vi "GUI BPM RMS Min Max Monitoring Graph Window.vi"() -> ()   [LabVIEW 2011, in "User Interface Window VIs.lvlib"]
uses:
  User Interface Window VIs.lvlib
  Types Definitions/Type Monitoring Sample.ctl
  <vilib>/Platform/TimedLoop/XDataNode/timing_clust.ctl
  <vilib>/Platform/TimedLoop/XDataNode/nitl_modes.ctl
  <vilib>/Platform/TimedLoop/XDataNode/wakeup.ctl
  <vilib>/Analysis/5stat.llb/RMS (DBL).vi
  <vilib>/express/express shared/transition.llb/Dynamic To Waveform Array.vi
  <vilib>/express/express signal manip/GetorSetDDTAttributes/Set DDT Attributes/SetT0.vi
  <vilib>/express/express shared/transition.llb/Waveform Array To Dynamic.vi
  <vilib>/Platform/TimedLoop/XDataNode/XDataNode.xnode
  <vilib>/express/express signal manip/GetorSetDDTAttributes/Set DDT Attributes/Set DDT Properties.xnode
  <vilib>/Analysis/NI_AALPro.lvlib
  <vilib>/Platform/TimedLoop/XDataNode/XDNodeRunTimeDep.lvlib
  Type Definitions.lvlib
panel:
  out "Time Stamp on FOFB Controller":timestamp caption="Data/Hora Atual no\nControlador do FOFB"
  in  "All/None":bool=TRUE caption="Todos/Nenhum"
  out "Graph":dynamicdata(graph)=[{"t0"=timestamp(3442305362.414053 s since 1904-01-01), "dt"=1.0, "Y"=[0.6809232435425464], "attributes"=variant("NI_ExpTimeStamp"=variant(timestamp timestamp(3442305362.414053 s since 1904-01-01)))}, {"t0"=timestamp(3442305362.414053 s since 1904-01-01), "dt"=1.0, "Y"=[1.8957212522578981], "attributes"=variant("NI_ExpTimeStamp"=variant(timestamp timestamp(3442305362.414053 s since 1904-01-01)))}, {"t0"=timestamp(3442305362.414053 s since 1904-01-01), "dt"=1.0, "Y"=[0.04856006519213252], "attributes"=variant("NI_ExpTimeStamp"=variant(timestamp timestamp(3442305362.414053 s since 1904-01-01)))}, {"t0"=timestamp(3442305362.414053 s since 1904-01-01), "dt"=1.0, "Y"=[0.5450159966663619], "attributes"=variant("NI_ExpTimeStamp"=variant(timestamp timestamp(3442305362.414053 s since 1904-01-01)))}, {"t0"=timestamp(3442305362.414053 s since 1904-01-01), "dt"=1.0, "Y"=[1.4720034670901994], "attributes"=variant("NI_ExpTimeStamp"=variant(timestamp timestamp(3442305362.414053 s since 1904-01-01)))}, {"t0"=timestamp(3442305362.414053 s since 1904-01-01), "dt"=1.0, "Y"=[0.0014319434180204427], "attributes"=variant("NI_ExpTimeStamp"=variant(timestamp timestamp(3442305362.414053 s since 1904-01-01)))}]
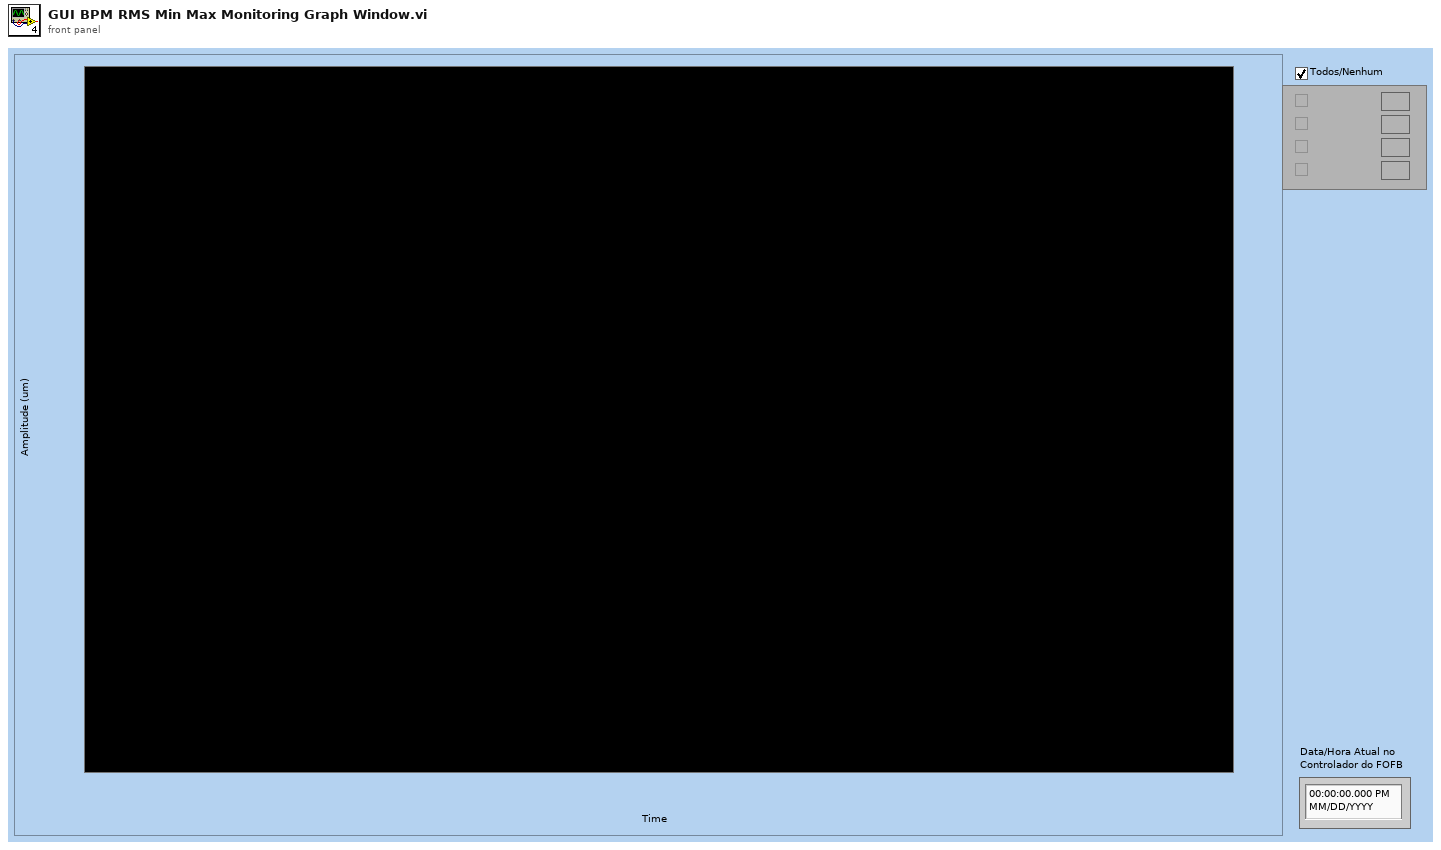
[diagram p1: front panel]
types:
  T1 = typedef "Type Definitions.lvlib/Type Monitoring Sample.ctl" = cluster{"Timestamp":timestamp, "Sample":dbl[]}
  T2 = typedef "XDNodeRunTimeDep.lvlib/timing_clust.ctl" = cluster{"Expected End [f-1]":u64, "Actual End [f-1]":u64, "Finished Late? [f-1]":bool, "Expected End [i-1]":u64, "Actual End [i-1]":u64, "Finished Late? [i-1]":bool, "Expected Start [i]":u64, "Actual Start [i]":u64, "Expected Start [f]":u64, "Actual Start [f]":u64, "Source Name":string, "Structure Name":string, "Period":i64, "Deadline":i64, "Offset":i64, "Start":i64, "Priority":i32, "Timeout":i32, "Mode":T3, "Wakeup Reason":T4, "Error":errorcluster, "Source Type":string, "Secondary Source Type":string, "Global End Time":u64, "Global Start Time":u64, "Frame Duration":u64, "Iteration Duration":u64, "Assigned CPU":i32, "I/O Scan Engine Mode":u32}
  T3 = typedef "XDNodeRunTimeDep.lvlib/nitl_modes.ctl" = enum32{"No Change", "Process missed periods, maintain original phase", "Discard missed periods, maintain original phase", "Process missed periods, ignore original phase", "Discard missed periods, ignore original phase"}
  T4 = typedef "XDNodeRunTimeDep.lvlib/wakeup.ctl" = enum32{"Normal", "Aborted", "Asynchronous wakeup", "Timing source error", "Timed loop error", "Timeout"}
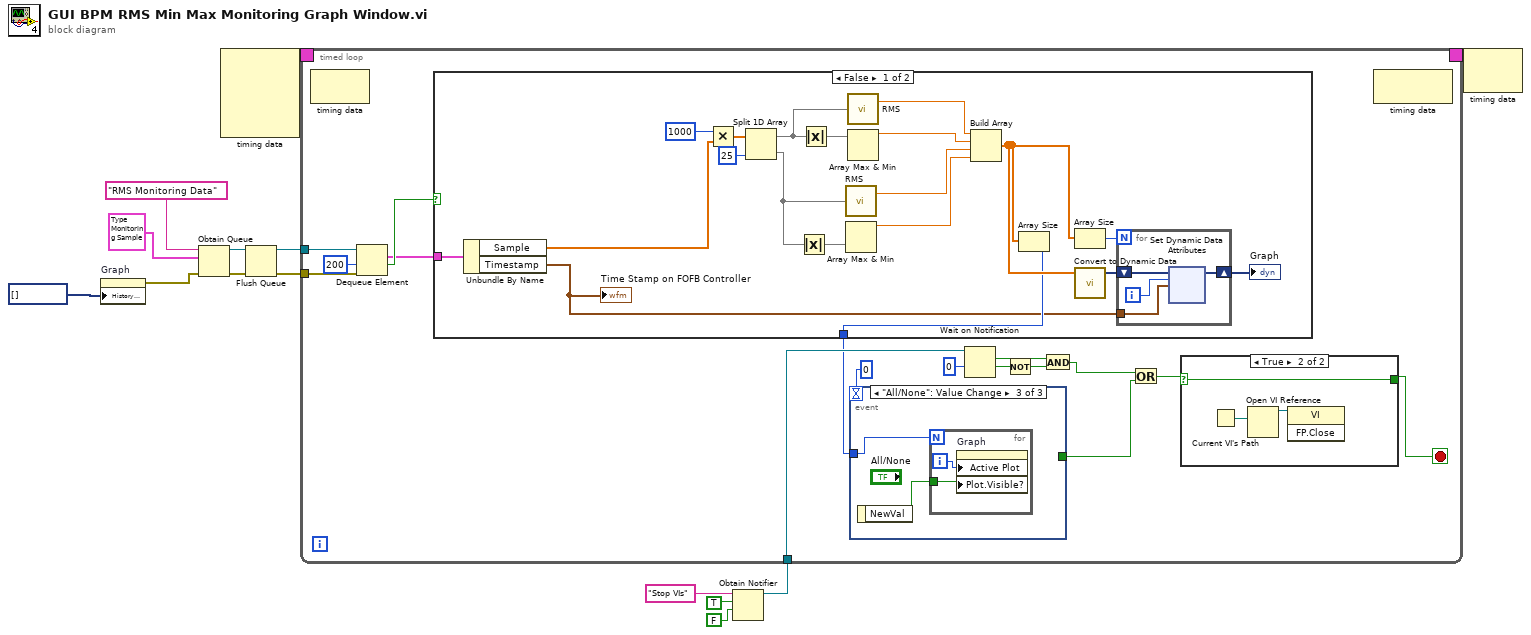
[diagram p0: block diagram]
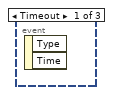
[diagram p4: hidden frame]
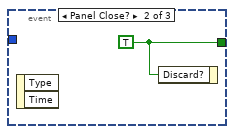
[diagram p5: hidden frame]
diagram:
  n1 = property on="Graph" class="WFChart (strict)"("History Data"=dynamicdata[] []) -> (error out=w5:errorcluster)  [unwired: 2 in, 1 out]
  n2 = Obtain Queue(name (unnamed)="RMS Monitoring Data", element data type=T1 {"Timestamp"=timestamp(0 s since 1904-01-01), "Sample"=[]} ("Monitoring Sample"), error in (no error)=w5) -> (queue out=w1:refnum<queue>, error out=w4:errorcluster)  [unwired: 2 in, 1 out]
  n3 = node-c288() -> (w14:T2)  [unwired: 4 in]
  n4 = Flush Queue(queue=w1, error in (no error)=w4) -> (queue out=w2:refnum<queue>, error out=w3:errorcluster)  [unwired: 1 out]
  n5 = Obtain Notifier(name (unnamed)="Stop VIs", notification data type=TRUE, create if not found? (T)=FALSE) -> (notifier out=w7:refnum<notifier>)  [unwired: 1 in, 2 out]
  n6 = timed-loop {
    timing: w14 -> [_]
    timing-out: [_] -> w13
    tunnel: w2 -> [w21]
    tunnel: w3 -> [w20]
    tunnel: w7 -> [w18]
    stop <- w22 stop-if-true
    n7 = node-c288() -> ()  [unwired: 1 in, 1 out]
    n8 = Dequeue Element(queue=w21, timeout in ms (-1)=200, error in (no error)=w20) -> (element=w15:T1, timed out?=w16:bool)  [unwired: 2 out]
    n9 = case shown="False" w16 {
      tunnel: [w34 _] -> w17
      tunnel: w15 -> [w33 _]
      frame False {
        n10 = Unbundle By Name(w33) -> ("Sample"=w32:dbl[], "Timestamp"=w31:timestamp)
        "Time Stamp on FOFB Controller" <- w31
        n11 = Multiply(x=1000, y=w32) -> (x*y=w39:dbl[])
        n12 = Split 1D Array(array=w39, index=25) -> (first subarray=w38:dbl[], second subarray=w37:dbl[])
        n13 = Absolute Value(x=w37) -> (abs(x)=w42:dbl[])
        n14 = Absolute Value(x=w38) -> (abs(x)=w43:dbl[])
        n15 = call-poly <vilib>:"RMS.vi"("X"=w37) -> ("rms value"=w41:dbl)  [unwired: 1 out]
        n16 = Array Max & Min(array=w42) -> (max value=w40:dbl)  [unwired: 3 out]
        n17 = call-poly <vilib>:"RMS.vi"("X"=w38) -> ("rms value"=w46:dbl)  [unwired: 1 out]
        n18 = Array Max & Min(array=w43) -> (max value=w45:dbl)  [unwired: 3 out]
        n19 = Build Array(w46, w45, w41, w40) -> (w35:dbl[])
        n20 = Array Size(array=w35) -> (size(s)=w34:i32)
        n21 = Array Size(array=w35) -> (size(s)=w49:i32)
        n22 = call "Convert to Dynamic Data"("Array"=w35) -> ("Dynamic Data Type"=w48:dynamicdata)  [unwired: 3 in]
        n23 = for {
          N: w49 -> [_]
          shift-right: [w53] -> w47
          shift-left: w48 -> [w51]
          tunnel: w31 -> [w50]
          i -> [w52]
          n24 = xnode ("Set Dynamic Data Attributes")("Signals In"=w51, "Signal Index"=w52, "Timestamp"=w50) -> ("Signals Out"=w53:dynamicdata)  [unwired: 1 in, 1 out]
        }
        "Graph" <- w47
      }
      frame True {
      }
    }
    n25 = event shown="[2] \"All/None\": Value Change" {
      selector: _ -> [_ _ _]
      dyn-events: _ -> [_ _ _]
      timeout: 0 -> [_ _ _]
      tunnel: [_ w71 _] -> w29
      tunnel: w17 -> [_ _ w72]
      event Timeout {
        n26 = event-data() -> ()  [unwired: 1 in, 2 out]
      }
      event Panel Close? {
        w71 = TRUE
        n27 = event-data() -> ()  [unwired: 1 in, 2 out]
        n28 = event-data("Discard?"=w71) -> ()  [unwired: 1 in, 1 out]
      }
      event "All/None": Value Change {
        n29 = event-data() -> ("NewVal"=w73:bool)  [unwired: 1 in]
        n30 = for {
          N: w72 -> [_]
          tunnel: w73 -> [w75]
          i -> [w74]
          n31 = property on="Graph" class="WFChart (strict)"("Active Plot"=w74, "Plot.Visible?"=w75) -> ()  [unwired: 2 in, 2 out]
        }
      }
    }
    n32 = Wait on Notification(notifier=w18, timeout in ms (-1)=0) -> (notification=w28:bool, timed out?=w26:bool)  [unwired: 2 in, 2 out]
    n33 = Not(x=w26) -> (.not. x?=w27:bool)
    n34 = And(x=w28, y=w27) -> (x .and. y?=w24:bool)
    n35 = Or(x=w24, y=w29) -> (x .or. y?=w23:bool)
    n36 = case shown="True" w23 {
      selector: w23 -> [w67 w69]
      tunnel: [w67 w69] -> w22
      frame False {
      }
      frame True {
        n37 = Current VI's Path() -> (path=w68:path)
        n38 = Open VI Reference(vi path=w68) -> (vi reference=w70:refnum<vi>)  [unwired: 5 in, 1 out]
        n39 = invoke class="VI" method="FP.Close"(reference=w70) -> ()  [unwired: 2 in, 3 out]
      }
    }
    n40 = node-c288() -> ()  [unwired: 1 in, 1 out]
  }
  n41 = node-c288(w13) -> ()  [unwired: 1 out]
